vi "精切.vi"() -> ()   [LabVIEW 2014]
panel:
  out "精切项目":string
  out "精切上料车条码":string
  out "精切下料车条码":string
  out "精切当前状态":string
  out "精切工位生产信息":string[][](table)
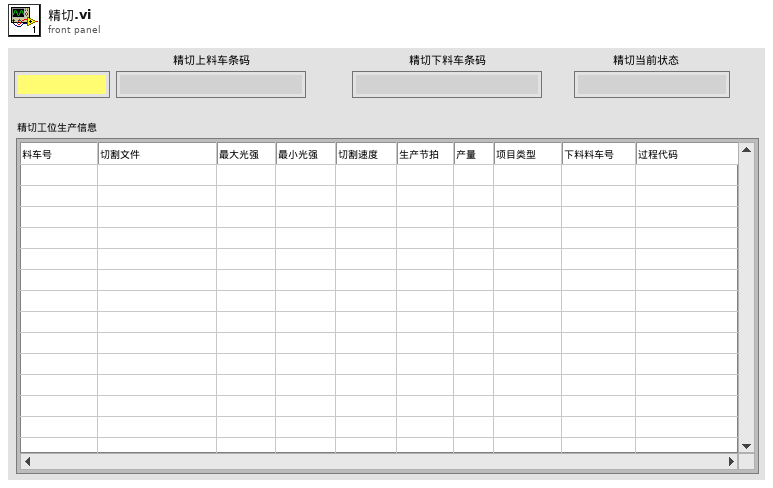
[diagram p1: front panel]
types:
  T1 = cluster{"精切工位生产信息":refnum<vi>, "精切上料车条码":refnum<vi>, "精切当前状态":refnum<vi>, "精切下料车条码":refnum<vi>, "精切项目":refnum<vi>}
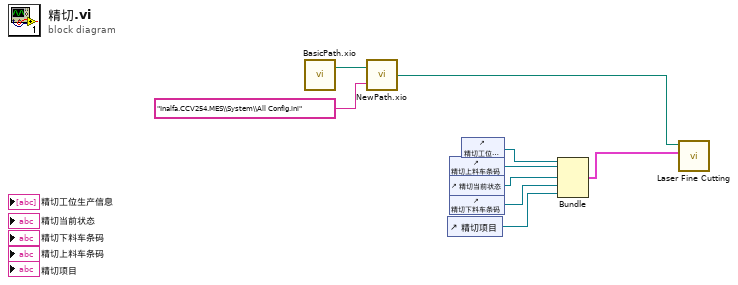
[diagram p0: block diagram]
diagram:
  n1 = call "BasicPath.xio.vi"() -> ("stripped path"=w8:path)  [unwired: 1 in, 1 out]
  n2 = call "NewPath.xio.vi"("Append path"="Inalfa.CCV254.MES\\System\\All Config.ini", "Basic path"=w8) -> ("New path"=w7:path)
  n3 = control-ref of="精切项目"() -> (w2:refnum<vi>)
  n4 = control-ref of="精切上料车条码"() -> (w6:refnum<vi>)
  n5 = control-ref of="精切当前状态"() -> (w5:refnum<vi>)
  n6 = control-ref of="精切下料车条码"() -> (w4:refnum<vi>)
  n7 = control-ref of="精切工位生产信息"() -> (w3:refnum<vi>)
  n8 = Bundle("精切工位生产信息"=w3, "精切上料车条码"=w6, "精切当前状态"=w5, "精切下料车条码"=w4, "精切项目"=w2) -> (w1:T1)  [unwired: 1 in]
  n9 = call "Laser Fine Cutting.vi"("configuration file path"=w7, "fine cutting msic"=w1) -> ()  [unwired: 4 in]
